vi "SIM RK Fixed Coefficients.vi"(1 "continuous integrator":T1=enum."RK 23") -> (0 "Runga-Kutte data out":T2={"weighting coefficients"=[[0.5, 0.0, 0.0, 0.0], [0.0, 0.5, 0.0, 0.0], [0.0, 0.0, 1.0, 0.0], [0.16666666666666696, 0.3333333333333333, 0.3333333333333333, 0.16666666666666666]], "time step fractions"=[0.5, 0.5, 1.0, 1.0], "Number of sub steps"=3} {"time step fractions" format="%.5f"; "weighting coefficients" format="%.5f"})   [LabVIEW 2018]
uses:
  SIM Runga-Kutte data - fixed step.ctl
  SIM integration method.ctl
panel:
  in  "Runga-Kutte data Euler 1":T2={"weighting coefficients"=[[1.0]], "time step fractions"=[1.0], "Number of sub steps"=1} {"time step fractions" format="%.5f"; "weighting coefficients" format="%.5f"}
  in  "Runga-Kutte data \"Trapezoid\" 2":T2={"weighting coefficients"=[[1.0, 0.0], [0.5, 0.5]], "time step fractions"=[1.0, 1.0], "Number of sub steps"=2} {"time step fractions" format="%.5f"; "weighting coefficients" format="%.5f"}
  in  "Runga-Kutte data Ralston 3":T2={"weighting coefficients"=[[0.5, 0.0, 0.0], [0.0, 0.75, 0.0], [0.2222222222222222, 0.3333333333333333, 0.4444444444444444]], "time step fractions"=[0.5, 0.75, 1.0], "Number of sub steps"=3} {"time step fractions" format="%.5f"; "weighting coefficients" format="%.5f"}
  in  "Runga-Kutte data classical 4":T2={"weighting coefficients"=[[0.5, 0.0, 0.0, 0.0], [0.0, 0.5, 0.0, 0.0], [0.0, 0.0, 1.0, 0.0], [0.16666666666666696, 0.3333333333333333, 0.3333333333333333, 0.16666666666666666]], "time step fractions"=[0.5, 0.5, 1.0, 1.0], "Number of sub steps"=4} {"time step fractions" format="%.5f"; "weighting coefficients" format="%.5f"}
  # "The last row of weighting coeff's is for the major step output\n(i.e. the coeff's below the line in the butcher array)"
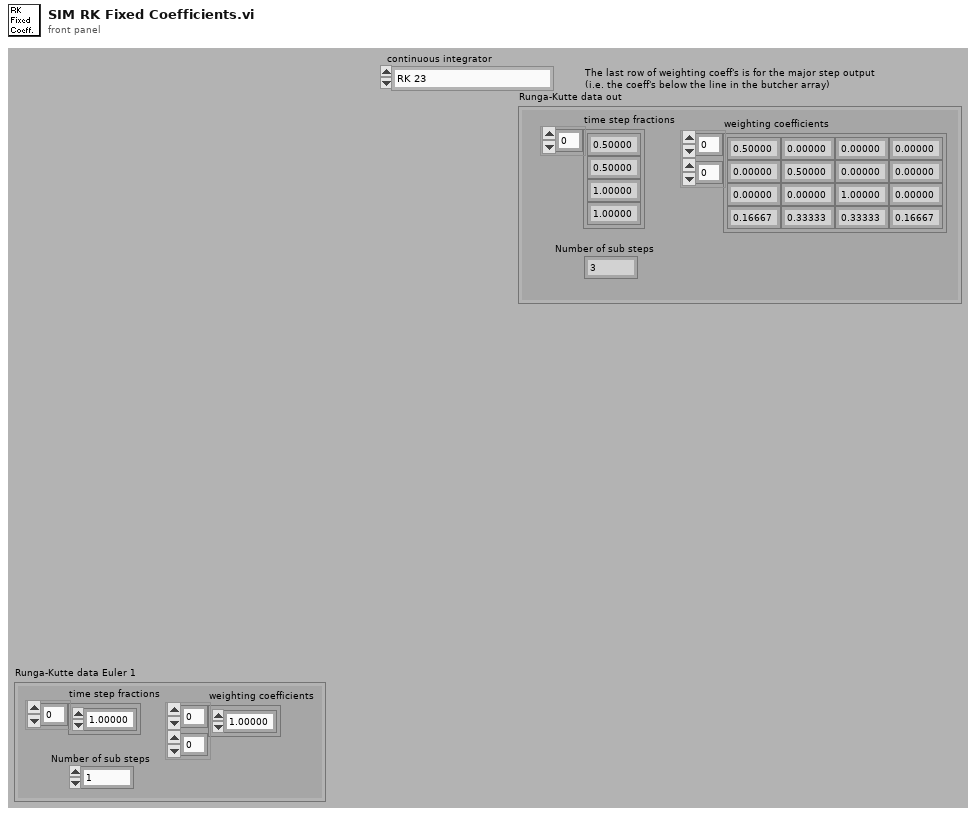
[diagram p1: front panel]
types:
  T1 = typedef "SIM integration method.ctl" = enum16{"RK 1 (Euler)", "Linearizer", "State Query", "Trim Eval", "Adams", "RK 3", "RK 4", "RK 45", "BDF", "RK 2", "RK 23", "Rosenbrock", "Discrete States Only"}
  T2 = typedef "SIM Runga-Kutte data - fixed step.ctl" = cluster{"weighting coefficients":dbl[][], "time step fractions":dbl[], "Number of sub steps":i32}
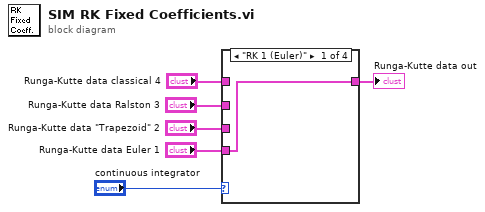
[diagram p0: block diagram]
diagram:
  n1 = case shown="\"RK 1 (Euler)\"" "continuous integrator" {
    tunnel: "Runga-Kutte data Euler 1" -> [w7 _ _ _]
    tunnel: "Runga-Kutte data \"Trapezoid\" 2" -> [_ w8 _ _]
    tunnel: "Runga-Kutte data Ralston 3" -> [_ _ w9 _]
    tunnel: "Runga-Kutte data classical 4" -> [_ _ _ w10]
    tunnel: [w7 w8 w9 w10] -> w1
    frame "RK 1 (Euler)" {
    }
    frame "RK 2" {
    }
    frame "RK 3" {
    }
    frame "RK 4", Default {
    }
  }
  "Runga-Kutte data out" <- w1
